vi "_lvVersion - lvproj.vi"(8 "error in (no error)":errorcluster, 11 "Path":path) -> (0 "error out":errorcluster, 2 "text":string, 3 "Path(dup)":path)   [LabVIEW 2014]
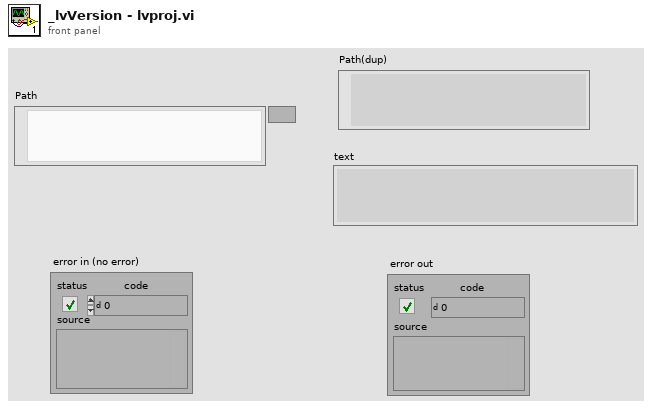
[diagram p1: front panel]
types:
  T1 = enum16{"open", "replace", "create", "open or create", "replace or create", "replace or create with confirmation"}
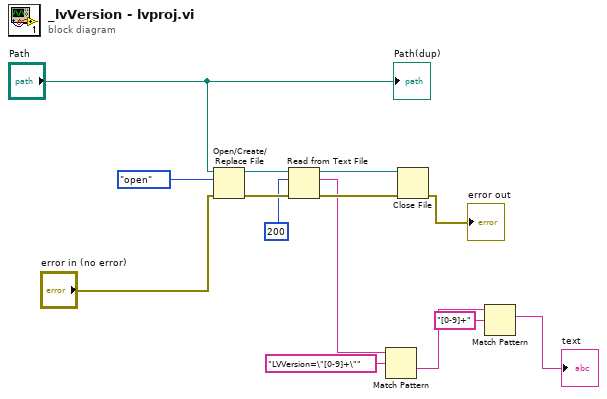
[diagram p0: block diagram]
diagram:
  n1 = Open/Create/Replace File(file path (use dialog)="Path", error in="error in (no error)", operation (0:open)=T1."open") -> (refnum out=w14:refnum<file>, error out=w12:errorcluster)  [unwired: 3 in, 1 out]
  n2 = Read from Text File(file (use dialog)=w14, count=200, error in=w12) -> (refnum out=w13:refnum<file>, text=w5:string, error out=w11:errorcluster)  [unwired: 1 in, 1 out]
  n3 = Match Pattern(string=w5, regular expression="LVVersion=\"[0-9]+\"") -> (match substring=w3:string)  [unwired: 1 in, 3 out]
  n4 = Close File(refnum=w13, error in=w11) -> (error out=→"error out":errorcluster)  [unwired: 1 out]
  n5 = Match Pattern(string=w3, regular expression="[0-9]+") -> (match substring=→"text":string)  [unwired: 1 in, 3 out]
  "Path(dup)" <- "Path"
